vi "Recipe_Line_Update.vi"(11 "Recipe_Board_Ref":refnum<vi>) -> (3 "Recipe_Index":i32)   [LabVIEW 2014]
panel:
  in  "Stop Button":bool
  in  "Tab Control":T1(tab)=enum."ACP"
  in  "Common":T2={"Center_Frequency(Hz)"=820000000.0, "Standard"=enum."CW", "Operation_Mode"=enum."PinSweep"} {"Center_Frequency(Hz)" format="%#_6p"}
  in  "Switch":cluster{"Switch_In":string, "Switch_Out":string}={"Switch_In"="ch3A", "Switch_Out"="ch3B"}
  in  "RFSG":T3={"RFSG_ExternalGain(dB)"=0.0, "RFSG_Pin_Start(dBm)"=-20.0, "RFSG_Pin_End(dBm)"=0.0, "Pin_Steps"=20.0} {"RFSG_ExternalGain(dB)" format="%#_6p"; "RFSG_Pin_Start(dBm)" format="%#_6p"; "RFSG_Pin_End(dBm)" format="%#_6p"; "Pin_Steps" format="%#_6p"}
  in  "RFSA":T4={"RFSA_Bandwidth(Hz)"=20000000.0, "RFSA_RBW(Hz)"=100000.0, "RFSA_ExternalAtten(dB)"=0.0} {"RFSA_ExternalAtten(dB)" format="%#_6p"; "RFSA_RBW(Hz)" format="%#_6p"; "RFSA_Bandwidth(Hz)" format="%#_6p"}
  in  "DC":T5={"DC1_Start(V)"=3.4, "DC1_End(V)"=3.4, "DC1_Steps"=1.0, "DC2_Start(V)"=3.7, "DC2_End(V)"=3.7, "DC2_Steps"=1.0} {"DC2_Steps" format="%#_6p"; "DC2_End(V)" format="%#_6p"; "DC2_Start(V)" format="%#_6p"; "DC1_Steps" format="%#_6p"; "DC1_End(V)" format="%#_6p"; "DC1_Start(V)" format="%#_6p"}
  in  "ACP":T6={"Ref_Ch_Bandwidth(Hz)"=9000000.0, "Offset_Freq(Hz)"=[10000000.0, 7500000.0, 12500000.0], "Int_Bandwidth(Hz)"=[9000000.0, 3840000.0, 3840000.0]} {"Int_Bandwidth(Hz)" format="%#_6p"; "Offset_Freq(Hz)" format="%#_6p"; "Ref_Ch_Bandwidth(Hz)" format="%#_6p"}
  in  "OK Button":bool
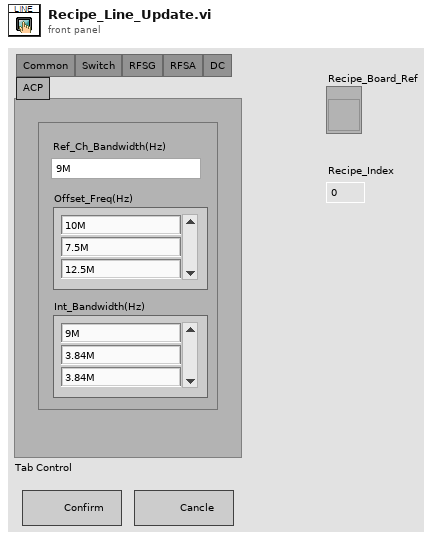
[diagram p1: front panel]
types:
  T1 = enum32{"Common", "Switch", "RFSG", "RFSA", "DC", "ACP"}
  T2 = cluster{"Center_Frequency(Hz)":dbl, "Standard":enum16{"CW", "LTE", "WCDMA", "GSM", "EDGE"}, "Operation_Mode":enum16{"PinSweep", "SingleMeasure"}}
  T3 = cluster{"RFSG_ExternalGain(dB)":dbl, "RFSG_Pin_Start(dBm)":dbl, "RFSG_Pin_End(dBm)":dbl, "Pin_Steps":dbl}
  T4 = cluster{"RFSA_Bandwidth(Hz)":dbl, "RFSA_RBW(Hz)":dbl, "RFSA_ExternalAtten(dB)":dbl}
  T5 = cluster{"DC1_Start(V)":dbl, "DC1_End(V)":dbl, "DC1_Steps":dbl, "DC2_Start(V)":dbl, "DC2_End(V)":dbl, "DC2_Steps":dbl}
  T6 = cluster{"Ref_Ch_Bandwidth(Hz)":dbl, "Offset_Freq(Hz)":dbl[], "Int_Bandwidth(Hz)":dbl[]}
  T7 = cluster{"Common":cluster{"Center_Frequency(Hz)":dbl, "Standard":enum16{"CW", "LTE", "WCDMA", "GSM", "EDGE"}, "Operation_Mode":enum16{"PinSweep", "SingleMeasure"}}, "Switch":cluster{"Switch_In":string, "Switch_Out":string}, "RFSG":cluster{"RFSG_ExternalGain(dB)":dbl, "RFSG_Pin_Start(dBm)":dbl, "RFSG_Pin_End(dBm)":dbl, "Pin_Steps":dbl}, "RFSA":cluster{"RFSA_Bandwidth(Hz)":dbl, "RFSA_RBW(Hz)":dbl, "RFSA_ExternalAtten(dB)":dbl}, "DC":cluster{"DC1_Start(V)":dbl, "DC1_End(V)":dbl, "DC1_Steps":dbl, "DC2_Start(V)":dbl, "DC2_End(V)":dbl, "DC2_Steps":dbl}, "ACP":cluster{"Ref_Ch_Bandwidth(Hz)":dbl, "Offset_Freq(Hz)":dbl[], "Int_Bandwidth(Hz)":dbl[]}}
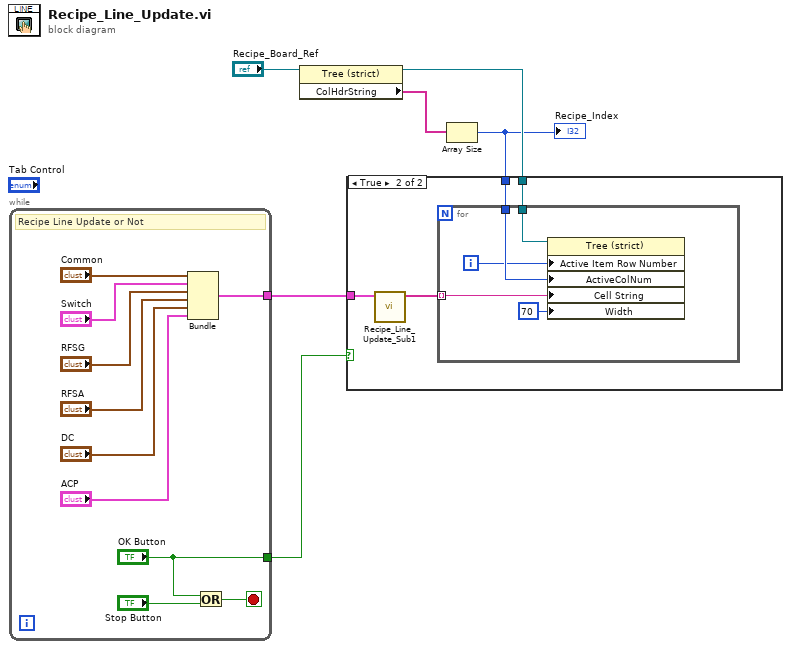
[diagram p0: block diagram]
diagram:
  n1 = while {
    tunnel: [w10] -> w4
    tunnel: ["OK Button"] -> w2
    stop <- w8 stop-if-true
    # "Recipe Line Update or Not"
    n2 = Bundle("Common"="Common", "Switch"="Switch", "RFSG"="RFSG", "RFSA"="RFSA", "DC"="DC", "ACP"="ACP") -> (w10:T7)  [unwired: 1 in]
    n3 = Or(x="OK Button", y="Stop Button") -> (x .or. y?=w8:bool)
  }
  n4 = property class="Tree (strict)"(reference="Recipe_Board_Ref") -> (reference out=w3:refnum<vi>, "ColHdrString"=w5:string[])  [unwired: 1 in, 1 out]
  n5 = Array Size(array=w5) -> (size(s)=w1:i32)
  "Recipe_Index" <- w1
  n6 = case shown="True" w2 {
    tunnel: w4 -> [_ w20]
    tunnel: w1 -> [_ w18]
    tunnel: w3 -> [_ w17]
    frame False {
    }
    frame True {
      n7 = call "Recipe_Line_Update_Sub1.vi"("Parameters"=w20) -> ("Parameter_str"=w19:string[])  [unwired: 10 in]
      n8 = for {
        tunnel: w19 -> [w25] mode=indexing
        tunnel: w18 -> [w23]
        tunnel: w17 -> [w24]
        i -> [w22]
        n9 = property class="Tree (strict)"(reference=w24, "Active Item Row Number"=w22, "ActiveColNum"=w23, "Cell String"=w25, "Width"=70 ("Active Cell:Cell Size:Width")) -> ()  [unwired: 1 in, 2 out]
      }
    }
  }
